vi "CRYWindow Init.vi"(11 "sAction":string) -> ()   [LabVIEW 2013]
uses:
  <vilib>/Utility/miscctls.llb/LVRectTypeDef.ctl
  CRYMain Sub Window Global.vi
panel:
  out "error out":errorcluster
  in  "error in (no error)":errorcluster
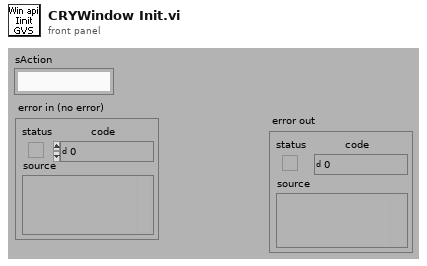
[diagram p1: front panel]
types:
  T1 = cluster{"VIName":string, "VI Refnum":refnum<vi>, "sDataID":string, "ObjectId":i16, "VITemp":string, "Width":i16, "Height":i16, "CapImg":bool, "IDDataView":i16}[]
  T2 = typedef "LVRectTypeDef.ctl" = cluster{"Left":i16, "Top":i16, "Right":i16, "Bottom":i16}
  T3 = cluster{"nID":i32[], "Frame":cluster{"nType":i32, "nParent":i32, "pVIW":refnum<vi>, "pSPW":refnum<vi>, "nTypeF":i32, "pVIF":refnum<vi>, "pSPF":refnum<vi>, "nIDSpliter":i32, "nProperty":i32, "Bound":T2, "nID":i32, "nData":i32, "sData":string, "pWVI":refnum<vi>, "sTitle":string, "cPages":cluster{"nPage":i32, "sTitle":string, "sIcon":string, "pVI":refnum<vi>, "nID":i32}[], "pTab":refnum<vi>, "nIDPages":i32[], "pSPT":refnum<vi>, "sTemp":string, "nDockID":i32, "nDockLR":i32, "sIcon":string}[]}
  T4 = cluster{"nID":i32[], "Spliter":cluster{"nType":i32, "nTypeP":i32, "pVI":refnum<vi>, "pSpliter":refnum<vi>, "pSPL":refnum<vi>, "pVIL":refnum<vi>, "pSPR":refnum<vi>, "pVIR":refnum<vi>, "nIDTL":i32, "nIDL":i32, "nIDTR":i32, "nIDR":i32, "nID":i32, "nIDParent":i32, "nData":i32, "sData":string}[]}
  T5 = cluster{"CLOSE_HIDE":i32, "CLOSE_CLOSE":i32, "DOCK_ENABLE":i32, "DOCK_DISABLE":i32, "FOCUS_SHOW":i32, "FOCUS_HIDE":i32}
  T6 = enum32{"Invalid", "Standard", "Closed", "Hidden", "Minimized", "Maximized"}
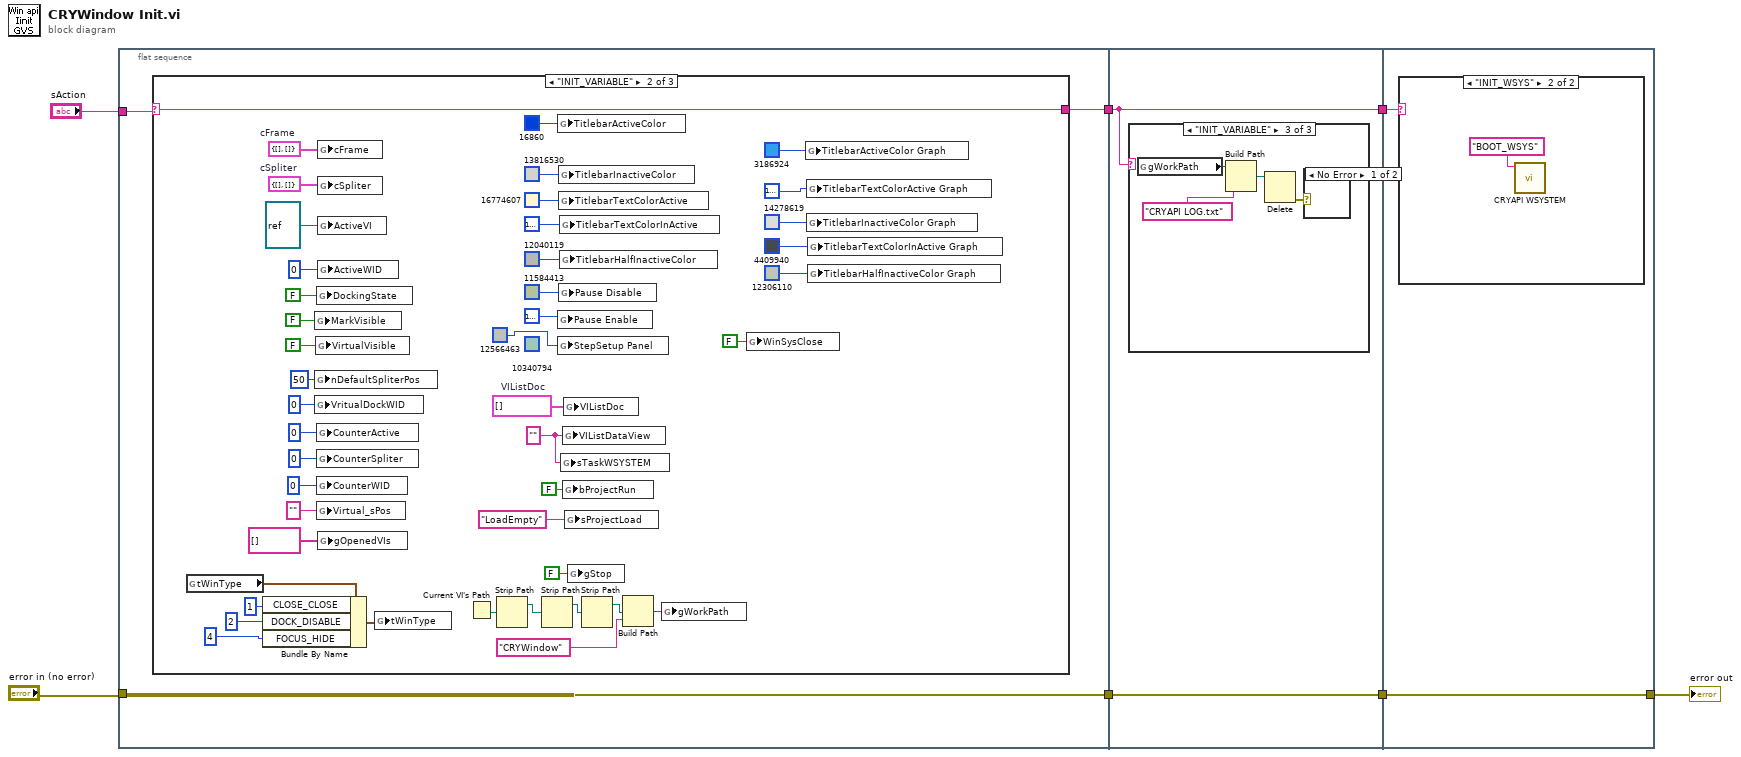
[diagram p0: block diagram]
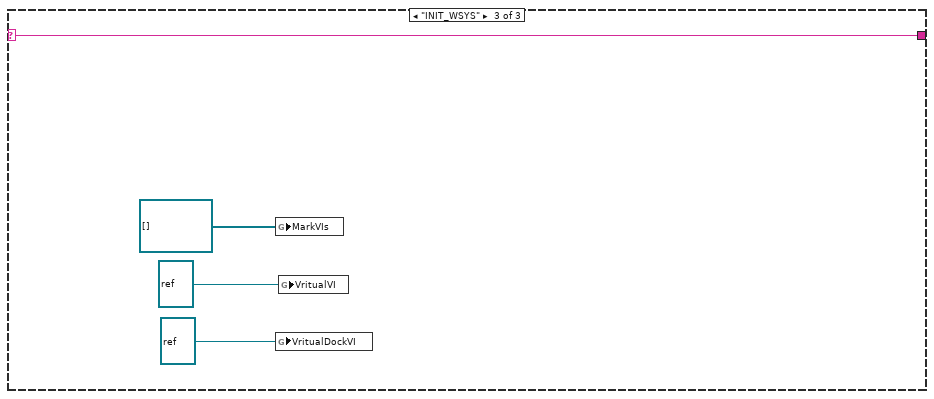
[diagram p3: hidden frame]
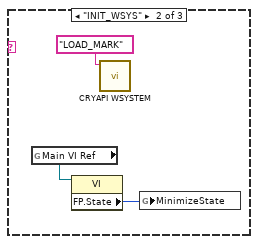
[diagram p5: hidden frame]
diagram:
  n1 = flat-sequence {
    tunnel: [w10] -> w5
    tunnel: [w8] -> w3
    tunnel: "sAction" -> [w9]
    tunnel: "error in (no error)" -> [w10]
    tunnel: w5 -> [w62]
    tunnel: [w62] -> w4
    tunnel: w3 -> [w61]
    tunnel: [w61] -> w2
    tunnel: [w71] -> w6
    tunnel: w4 -> [w71]
    tunnel: w2 -> [w70]
    frame #0 {
      n2 = case shown="\"INIT_VARIABLE\"" w9 {
        selector: w9 -> [w11 w31 w57]
        tunnel: [w11 w31 w57] -> w8
        frame Default {
        }
        frame "INIT_VARIABLE" {
          (unwired) u32 10340794
          w30 = "" ("VIListDataView")
          w38 = T1 []  # VIListDoc
          w42 = T3 {"nID"=[], "Frame"=[]}  # cFrame
          w48 = T4 {"nID"=[], "Spliter"=[]}  # cSpliter
          n3 = global read "CRYMain Sub Window Global.vi" "tWinType"() -> (w47:T5)
          n4 = Bundle By Name(cluster=w47, "CLOSE_CLOSE"=1, "DOCK_DISABLE"=2, "FOCUS_HIDE"=4) -> (w43:T5)
          n5 = global write "CRYMain Sub Window Global.vi" "MarkVisible"(FALSE ("Virtual VI State")) -> ()
          n6 = global write "CRYMain Sub Window Global.vi" "nDefaultSpliterPos"(50 ("ActiveWID")) -> ()
          n7 = global write "CRYMain Sub Window Global.vi" "VritualDockWID"(0 ("ActiveWID")) -> ()
          n8 = global write "CRYMain Sub Window Global.vi" "VirtualVisible"(FALSE ("Mark VI State")) -> ()
          n9 = global write "CRYMain Sub Window Global.vi" "DockingState"(FALSE ("Docking_State")) -> ()
          n10 = global write "CRYMain Sub Window Global.vi" "CounterActive"(0 ("ChainCounter")) -> ()
          n11 = global write "CRYMain Sub Window Global.vi" "CounterSpliter"(0 ("ChainCounter")) -> ()
          n12 = global write "CRYMain Sub Window Global.vi" "CounterWID"(0 ("CounterWID")) -> ()
          n13 = global write "CRYMain Sub Window Global.vi" "Virtual_sPos"("" ("Virtual_sPos")) -> ()
          n14 = global write "CRYMain Sub Window Global.vi" "cFrame"(w42) -> ()
          n15 = global write "CRYMain Sub Window Global.vi" "cSpliter"(w48) -> ()
          n16 = global write "CRYMain Sub Window Global.vi" "ActiveVI"(refnum<vi> refnum ("Active_VIRef")) -> ()
          n17 = global write "CRYMain Sub Window Global.vi" "ActiveWID"(0 ("ActiveWID")) -> ()
          n18 = global write "CRYMain Sub Window Global.vi" "gOpenedVIs"(string[] [] ("gOpenedVIs")) -> ()
          n19 = global write "CRYMain Sub Window Global.vi" "tWinType"(w43) -> ()
          n20 = Current VI's Path() -> (path=w33:path)
          n21 = Strip Path(path=w33) -> (stripped path=w32:path)  [unwired: 1 out]
          n22 = Strip Path(path=w32) -> (stripped path=w34:path)  [unwired: 1 out]
          n23 = global write "CRYMain Sub Window Global.vi" "TitlebarActiveColor"(u32 16860 ("TitlebarActive")) -> ()
          n24 = global write "CRYMain Sub Window Global.vi" "Pause Enable"(u32 16777226) -> ()
          n25 = global write "CRYMain Sub Window Global.vi" "StepSetup Panel"(u32 12566463) -> ()
          n26 = global write "CRYMain Sub Window Global.vi" "TitlebarInactiveColor"(u32 13816530 ("TitlebarInActive")) -> ()
          n27 = global write "CRYMain Sub Window Global.vi" "TitlebarTextColorActive"(u32 16774607 ("TextColorActive")) -> ()
          n28 = global write "CRYMain Sub Window Global.vi" "Pause Disable"(u32 11584413) -> ()
          n29 = global write "CRYMain Sub Window Global.vi" "TitlebarTextColorInActive"(u32 16777222 ("TextColorInActive")) -> ()
          n30 = global write "CRYMain Sub Window Global.vi" "TitlebarHalfInactiveColor"(u32 12040119 ("TitlebarHalfInActive")) -> ()
          n31 = global write "CRYMain Sub Window Global.vi" "sTaskWSYSTEM"(w30) -> ()
          n32 = global write "CRYMain Sub Window Global.vi" "VIListDataView"(w30) -> ()
          n33 = global write "CRYMain Sub Window Global.vi" "bProjectRun"(FALSE ("bProjectRun")) -> ()
          n34 = global write "CRYMain Sub Window Global.vi" "VIListDoc"(w38) -> ()
          n35 = global write "CRYMain Sub Window Global.vi" "sProjectLoad"("LoadEmpty" ("sProjectLoad")) -> ()
          n36 = global write "CRYMain Sub Window Global.vi" "gStop"(FALSE ("gStop")) -> ()
          n37 = Strip Path(path=w34) -> (stripped path=w35:path)  [unwired: 1 out]
          n38 = Build Path(base path=w35, name or relative path="CRYWindow" ("name")) -> (appended path=w37:path)
          n39 = global write "CRYMain Sub Window Global.vi" "gWorkPath"(w37) -> ()
          n40 = global write "CRYMain Sub Window Global.vi" "WinSysClose"(FALSE ("WinSysClose")) -> ()
          n41 = global write "CRYMain Sub Window Global.vi" "TitlebarActiveColor Graph"(u32 3186924 ("TitlebarActiveColor Graph")) -> ()
          n42 = global write "CRYMain Sub Window Global.vi" "TitlebarTextColorActive Graph"(u32 16777226 ("TextColorActive")) -> ()
          n43 = global write "CRYMain Sub Window Global.vi" "TitlebarInactiveColor Graph"(u32 14278619 ("TextColorActive")) -> ()
          n44 = global write "CRYMain Sub Window Global.vi" "TitlebarTextColorInActive Graph"(u32 4409940 ("TextColorInActive")) -> ()
          n45 = global write "CRYMain Sub Window Global.vi" "TitlebarHalfInactiveColor Graph"(u32 12306110 ("TitlebarHalfInActive")) -> ()
        }
        frame "INIT_WSYS" {
          n46 = global write "CRYMain Sub Window Global.vi" "MarkVIs"(refnum<vi>[] [] ("MarkVI")) -> ()
          n47 = global write "CRYMain Sub Window Global.vi" "VritualDockVI"(refnum<vi> refnum ("Active_VIRef")) -> ()
          n48 = global write "CRYMain Sub Window Global.vi" "VritualVI"(refnum<vi> refnum ("Active_VIRef")) -> ()
        }
      }
    }
    frame #1 {
      n49 = case shown="\"INIT_VARIABLE\"" w61 {
        frame Default {
        }
        frame "INIT_WSYS" {
          n50 = global read "CRYMain Sub Window Global.vi" "Main VI Ref"() -> (w64:refnum<vi>)
          n51 = property class="VI"(reference=w64) -> ("FP.State"=w65:T6)  [unwired: 1 in, 2 out]
          n52 = call "CRYAPI WSYSTEM.vi"("sAction"="LOAD_MARK") -> ()  [unwired: 3 in, 8 out]
          n53 = global write "CRYMain Sub Window Global.vi" "MinimizeState"(w65) -> ()
        }
        frame "INIT_VARIABLE" {
          n54 = global read "CRYMain Sub Window Global.vi" "gWorkPath"() -> (w66:path)
          n55 = Build Path(base path=w66, name or relative path="CRYAPI LOG.txt" ("name")) -> (appended path=w68:path)
          n56 = Delete(path (use dialog)=w68) -> (error out=w67:errorcluster)  [unwired: 1 in, 5 out]
          n57 = case shown="No Error" w67 {
            frame No Error {
            }
            frame Error {
            }
          }
        }
      }
    }
    frame #2 {
      n58 = case shown="\"INIT_WSYS\"" w70 {
        frame Default {
        }
        frame "INIT_WSYS" {
          n59 = call "CRYAPI WSYSTEM.vi"("sAction"="BOOT_WSYS") -> ()  [unwired: 3 in, 8 out]
        }
      }
    }
  }
  "error out" <- w6
